vi "8channel_ADS_int_parser.vi"(11 "String in":string) -> (1 "Leftover":string, 2 "Stat":string, 3 "Data out":T1)   [LabVIEW 2023]
uses:
  <vilib>/Utility/error.llb/whitespace.ctl
  <vilib>/Utility/error.llb/Trim Whitespace One-Sided.vi
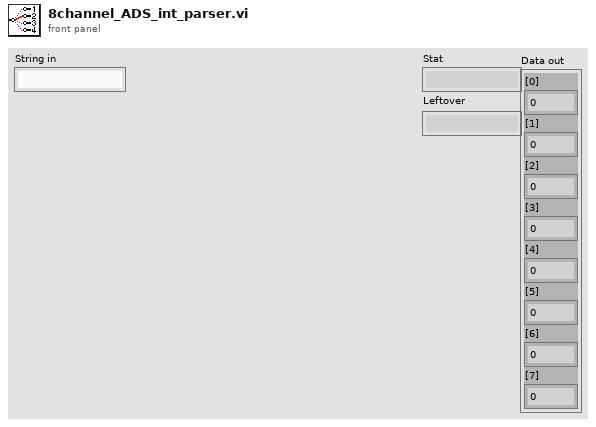
[diagram p1: front panel]
types:
  T1 = cluster{"[0]":dbl, "[1]":dbl, "[2]":dbl, "[3]":dbl, "[4]":dbl, "[5]":dbl, "[6]":dbl, "[7]":dbl}
  T2 = typedef "whitespace.ctl" = u16
  T3 = cluster{"String in":string, "String in":string, "String in":string, "String in":string, "String in":string, "String in":string, "String in":string, "String in":string}
  T4 = cluster{"String in":u32, "String in":u32, "String in":u32, "String in":u32, "String in":u32, "String in":u32, "String in":u32, "String in":u32}
  T5 = cluster{"String in":i32, "String in":i32, "String in":i32, "String in":i32, "String in":i32, "String in":i32, "String in":i32, "String in":i32}
  T6 = cluster{"String in":dbl, "String in":dbl, "String in":dbl, "String in":dbl, "String in":dbl, "String in":dbl, "String in":dbl, "String in":dbl}
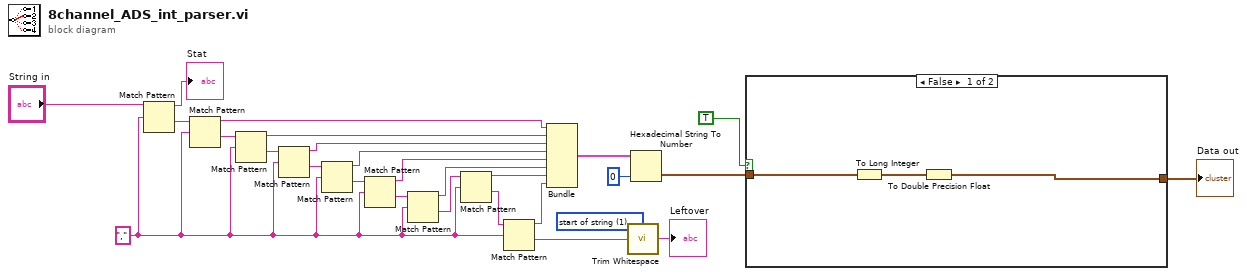
[diagram p0: block diagram]
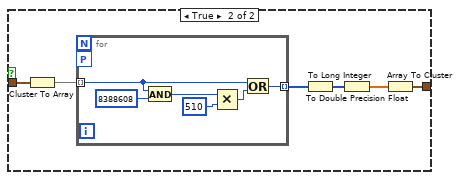
[diagram p2: hidden frame]
diagram:
  w5 = T2 1 items=["both", "start of string", "end of string"] ("location (both)")
  w18 = "," ("regular expression")
  n1 = Match Pattern(string="String in", regular expression=w18) -> (before substring=→"Stat":string, after substring=w25:string)  [unwired: 1 in, 2 out]
  n2 = Match Pattern(string=w25, regular expression=w18) -> (before substring=w17:string, after substring=w27:string)  [unwired: 1 in, 2 out]
  n3 = Match Pattern(string=w27, regular expression=w18) -> (before substring=w16:string, after substring=w24:string)  [unwired: 1 in, 2 out]
  n4 = Match Pattern(string=w24, regular expression=w18) -> (before substring=w15:string, after substring=w23:string)  [unwired: 1 in, 2 out]
  n5 = Match Pattern(string=w23, regular expression=w18) -> (before substring=w14:string, after substring=w22:string)  [unwired: 1 in, 2 out]
  n6 = Match Pattern(string=w22, regular expression=w18) -> (before substring=w13:string, after substring=w21:string)  [unwired: 1 in, 2 out]
  n7 = Match Pattern(string=w21, regular expression=w18) -> (before substring=w12:string, after substring=w20:string)  [unwired: 1 in, 2 out]
  n8 = Match Pattern(string=w20, regular expression=w18) -> (before substring=w11:string, after substring=w19:string)  [unwired: 1 in, 2 out]
  n9 = Match Pattern(string=w19, regular expression=w18) -> (before substring=w10:string, after substring=w6:string)  [unwired: 1 in, 2 out]
  n10 = Bundle("String in"=w17, "String in"=w16, "String in"=w15, "String in"=w14, "String in"=w13, "String in"=w12, "String in"=w11, "String in"=w10) -> (w8:T3)  [unwired: 1 in]
  n11 = call <vilib>:"Trim Whitespace.vi"("string"=w6, "location (both)"=w5) -> ("trimmed string"=→"Leftover":string)
  n12 = Hexadecimal String To Number(string=w8, default (0uL)=u32 0 ("default (0 U32)")) -> (number=w7:T4)  [unwired: 1 in, 1 out]
  n13 = case shown="False" TRUE {
    tunnel: w7 -> [w29 w36]
    tunnel: [w30 w34] -> w1
    frame False {
      n14 = To Long Integer(number=w29) -> (32bit integer=w28:T5)
      n15 = To Double Precision Float(number=w28) -> (double precision float=w30:T6)
    }
    frame True {
      n16 = Cluster To Array(cluster=w36) -> (array=w35:u32[])
      n17 = for {
        tunnel: w35 -> [w38] mode=indexing
        tunnel: [w37] -> w32 mode=indexing
        workers-P: _ -> [_]
        n18 = And(x=w38, y=8388608) -> (x .and. y?=w41:u32)
        n19 = Multiply(x=w41, y=510) -> (x*y=w40:u32)
        n20 = Or(x=w38, y=w40) -> (x .or. y?=w37:u32)
      }
      n21 = To Long Integer(number=w32) -> (32bit integer=w31:i32[])
      n22 = To Double Precision Float(number=w31) -> (double precision float=w33:dbl[])
      n23 = Array To Cluster(array=w33) -> (cluster=w34:T1)
    }
  }
  "Data out" <- w1
